vi "ETH2_E1A_Checksum.vi"(11 "Data":u8[](array[numeric])) -> (3 "Checksum 2":bool)   [LabVIEW 2022 SP3]
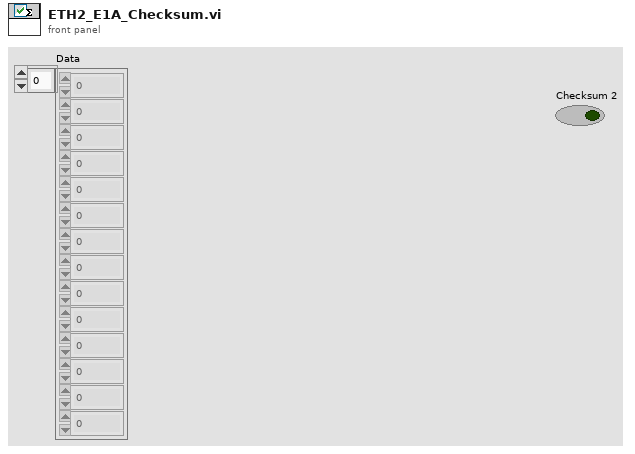
[diagram p1: front panel]
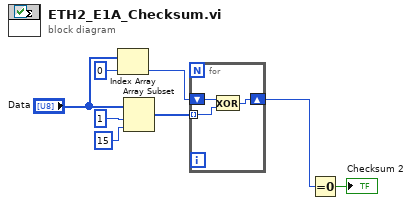
[diagram p0: block diagram]
diagram:
  n1 = Index Array(array="Data", index=0) -> (element=w6:u8)
  n2 = Array Subset(array="Data", index=1 ("length"), length=15 ("index")) -> (w7:u8[])
  n3 = for {
    shift-right: [w9] -> w1
    shift-left: w6 -> [w11]
    tunnel: w7 -> [w10] mode=indexing
    n4 = Exclusive Or(1:w10, 2:w11) -> (0:w9:u8)
  }
  n5 = Equal To 0?(x=w1) -> (x = 0?=→"Checksum 2":bool)
